vi "SUB_StimGenerator.vi"(0 "SampleNumIn":dbl, 1 "DataFromFile":T2(array[cluster]), 5 "PosInStimTable":i32, 6 "RelativeAmps":bool, 7 "StimType":string, 9 "StimTable":dbl[][](array[numeric]), 11 "UnitFactor":dbl, 12 "SampleRate":dbl, 14 "CommandDivider":dbl) -> (2 "unscaled wave":waveform(dbl), 3 "wave":waveform(dbl), 4 "Array":dbl[](array[numeric]), 10 "Holding":dbl, 13 "UnscaledArray":dbl[](array[numeric]), 15 "SampleNumOut":dbl)   [LabVIEW 2015]
uses:
  <vilib>/Analysis/1siggen.llb/Ramp Pattern by Samples.vi
  <vilib>/Analysis/NI_AALBase.lvlib
panel:
  out "SelCounter":i32
  in  "Cluster":T1={"Pattern"=0, "Mode"=0, "FrameN"=0, "SampleNum"=0, "Flags"=0, "SampleRate"=0.0, "Comment"="", "TimeStr"="", "Data"=[], "StimTable"=[], "NumInFile"=0, "PosInFile"=0, "TimeStamp"=timestamp(0 s since 1904-01-01), "RelAmp"=TRUE}
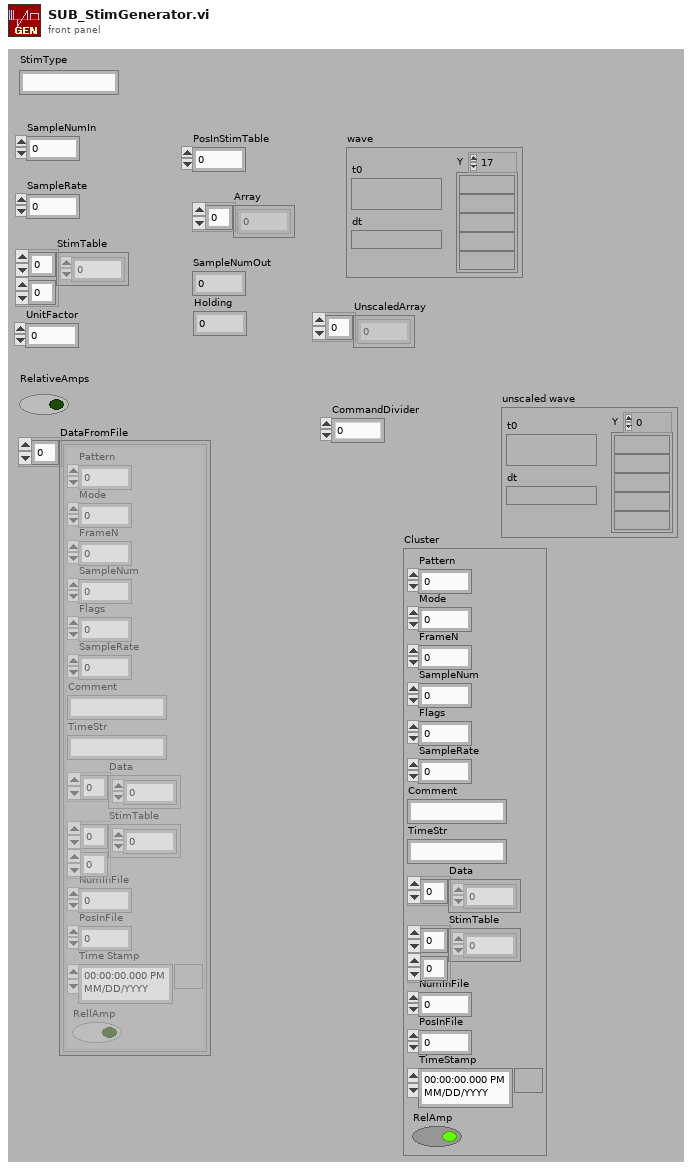
[diagram p1: front panel]
types:
  T1 = cluster{"Pattern":u8, "Mode":u8, "FrameN":u32, "SampleNum":u32, "Flags":u8, "SampleRate":dbl, "Comment":string, "TimeStr":string, "Data":dbl[], "StimTable":dbl[][], "NumInFile":i32, "PosInFile":i32, "TimeStamp":timestamp, "RelAmp":bool}
  T2 = cluster{"Pattern":u8, "Mode":u8, "FrameN":u32, "SampleNum":u32, "Flags":u8, "SampleRate":dbl, "Comment":string, "TimeStr":string, "Data":dbl[], "StimTable":dbl[][], "NumInFile":i32, "PosInFile":i32, "Time Stamp":timestamp, "RellAmp":bool}[]
  T3 = cluster{"Pattern":u8, "Mode":u8, "FrameN":u32, "SampleNum":u32, "Flags":u8, "SampleRate":dbl, "Comment":string, "TimeStr":string, "Data":dbl[], "StimTable":dbl[][], "NumInFile":i32, "PosInFile":i32, "Time Stamp":timestamp, "RellAmp":bool}
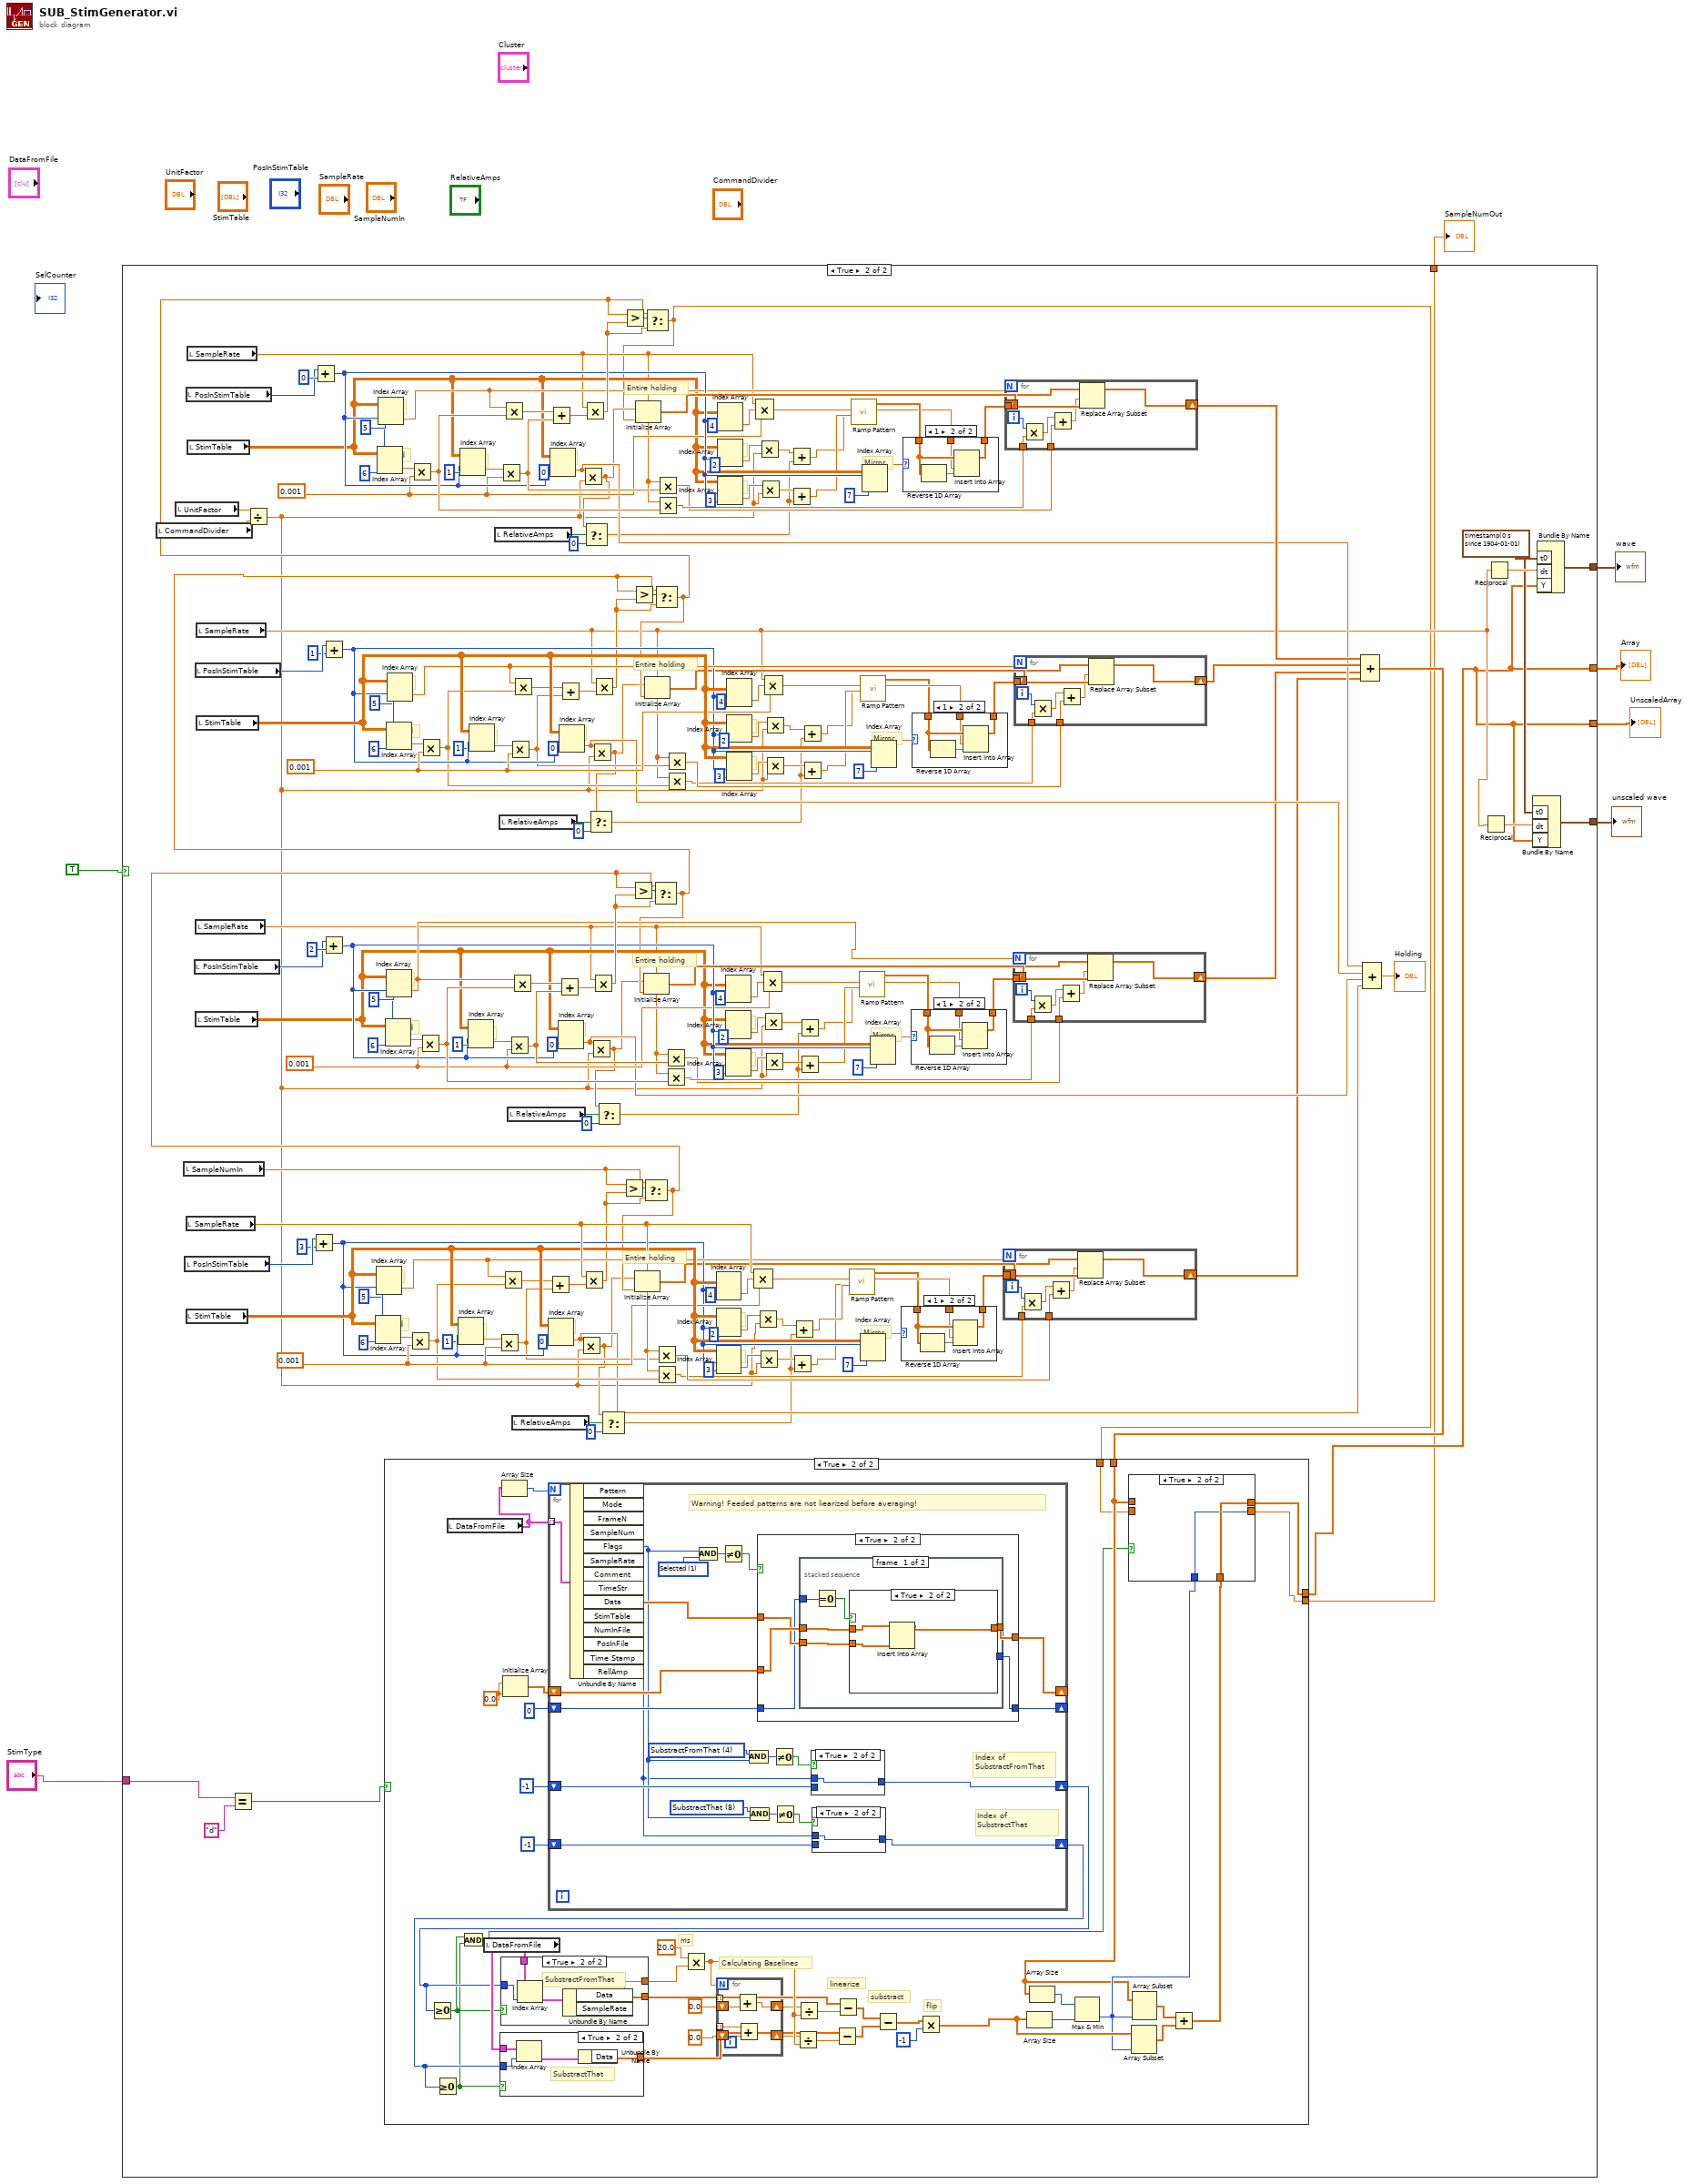
[diagram p0: block diagram]
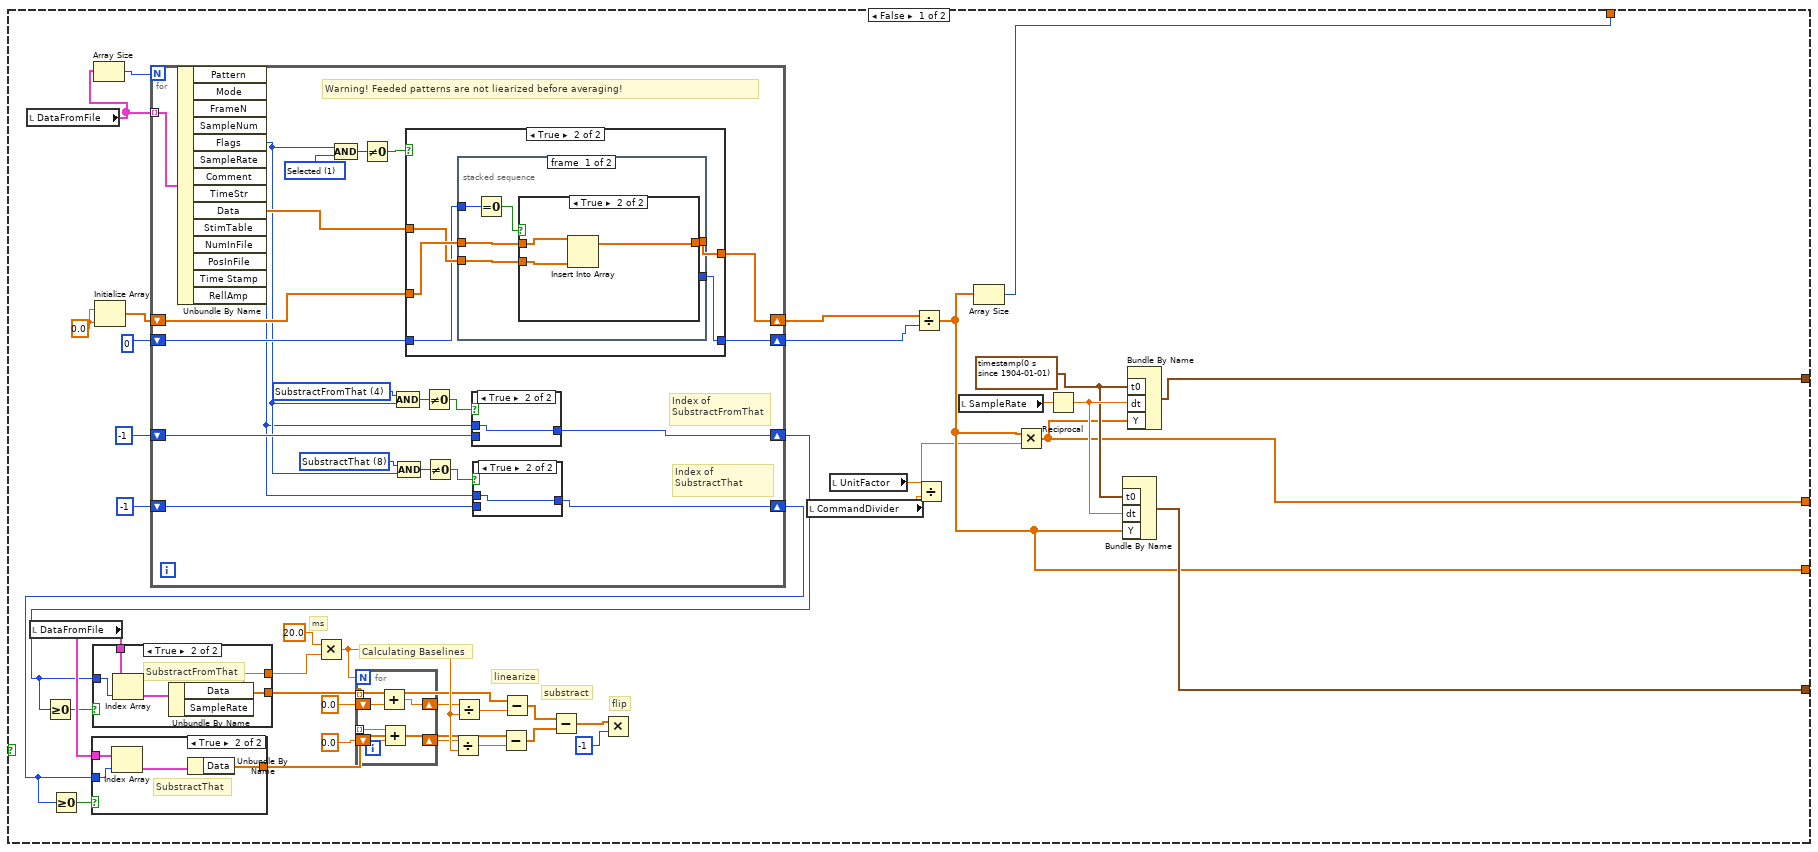
[diagram p2: hidden frame]
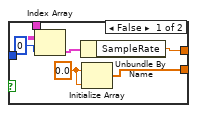
[diagram p3: hidden frame]
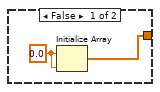
[diagram p4: hidden frame]
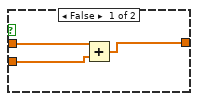
[diagram p8: hidden frame]
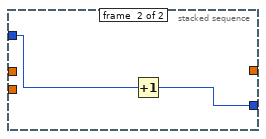
[diagram p9: hidden frame]
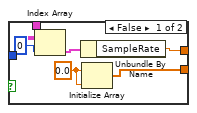
[diagram p12: hidden frame]
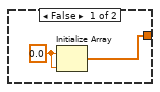
[diagram p13: hidden frame]
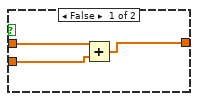
[diagram p17: hidden frame]
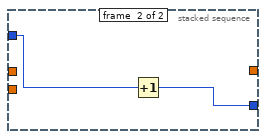
[diagram p18: hidden frame]
diagram:
  n1 = case shown="True" TRUE {
    tunnel: [w35 w119] -> w7
    tunnel: [w40 w130] -> w6
    tunnel: [w44 w129] -> w5
    tunnel: [w34 w121] -> w4
    tunnel: [w39 w121] -> w3
    tunnel: "StimType" -> [_ w116]
    frame False {
      w41 = timestamp(0 s since 1904-01-01)
      w47 = 0.0
      # "flip"
      # "substract"
      # "linearize"
      # "ms"
      # "Calculating Baselines"
      n2 = local read "DataFromFile"() -> (w37:T2)
      n3 = local read "DataFromFile"() -> (w28:T2)
      n4 = Array Size(array=w37) -> (size(s)=w38:i32)
      n5 = Initialize Array(w47, w47) -> (w46:dbl[])
      n6 = for {
        N: w38 -> [_]
        tunnel: w37 -> [w91] mode=indexing
        shift-right: [w85] -> w45
        shift-left: w46 -> [w87]
        shift-right: [w83] -> w36
        shift-left: 0 -> [w84]
        shift-right: [w79] -> w11
        shift-left: -1 -> [w78]
        shift-right: [w71] -> w9
        shift-left: -1 -> [w72]
        w76 = u16 8 items=["Selected"=1, "Deleted"=2, "SubstractFromThat"=4, "SubstractThat"=8] ("DataFrameFlags")
        w81 = u16 4 items=["Selected"=1, "Deleted"=2, "SubstractFromThat"=4, "SubstractThat"=8] ("DataFrameFlags")
        w90 = u16 1 items=["Selected"=1, "Deleted"=2, "Reserved1"=4, "Reserved2"=8] ("DataFrameFlags")
        # "Index of SubstractThat"
        # "Index of SubstractFromThat"
        # "Warning! Feeded patterns are not liearized before averaging!"
        n7 = Unbundle By Name(w91) -> ("Flags"=w74:u8, "Data"=w86:dbl[], "NumInFile"=w73:i32)  [unwired: 11 out]
        n8 = Compound Arithmetic op=AND(w74, w90) -> (w89:u16)
        n9 = Not Equal To 0?(x=w89) -> (x != 0?=w88:bool)
        n10 = Compound Arithmetic op=AND(w81, w74) -> (w82:u16)
        n11 = Compound Arithmetic op=AND(w76, w74) -> (w75:u16)
        n12 = case shown="True" w88 {
          tunnel: w87 -> [w97 w102]
          tunnel: [w97 w100] -> w85
          tunnel: w86 -> [_ w101]
          tunnel: w84 -> [w96 w99]
          tunnel: [w96 w98] -> w83
          frame False {
          }
          frame True {
            n13 = stacked-sequence {
              tunnel: w102 -> [w107 _]
              tunnel: w101 -> [w106 _]
              tunnel: [w105 _] -> w100
              tunnel: w99 -> [w103 w115]
              tunnel: [_ w114] -> w98
              frame #0 {
                n14 = Equal To 0?(x=w103) -> (x = 0?=w104:bool)
                n15 = case shown="True" w104 {
                  tunnel: w107 -> [w109 w112]
                  tunnel: w106 -> [w110 w111]
                  tunnel: [w108 w113] -> w105
                  frame False {
                    n16 = Add(x=w109, y=w110) -> (x+y=w108:dbl[])
                  }
                  frame True {
                    n17 = Insert Into Array(array=w112, new element=w111) -> (w113:dbl[])  [unwired: 1 in]
                  }
                }
              }
              frame #1 {
                n18 = Increment(x=w115) -> (x+1=w114:i32)
              }
            }
          }
        }
        n19 = Not Equal To 0?(x=w82) -> (x != 0?=w80:bool)
        n20 = Not Equal To 0?(x=w75) -> (x != 0?=w77:bool)
        n21 = case shown="True" w80 {
          tunnel: w73 -> [_ w95]
          tunnel: [w94 w95] -> w79
          tunnel: w78 -> [w94 _]
          frame False {
          }
          frame True {
          }
        }
        n22 = case shown="True" w77 {
          tunnel: w73 -> [_ w93]
          tunnel: [w92 w93] -> w71
          tunnel: w72 -> [w92 _]
          frame False {
          }
          frame True {
          }
        }
      }
      n23 = Greater Or Equal To 0?(x=w11) -> (x >= 0?=w12:bool)
      n24 = Greater Or Equal To 0?(x=w9) -> (x >= 0?=w10:bool)
      n25 = case shown="True" w10 {
        tunnel: w28 -> [_ w64]
        tunnel: w9 -> [_ w63]
        tunnel: [w59 w61] -> w17
        frame False {
          w60 = 0.0
          n26 = Initialize Array(w60, w60) -> (w59:dbl[])
        }
        frame True {
          # "SubstractThat"
          n27 = Index Array(array=w64, index=w63) -> (element=w62:T3)
          n28 = Unbundle By Name(w62) -> ("Data"=w61:dbl[])
        }
      }
      n29 = case shown="True" w12 {
        tunnel: w11 -> [_ w58]
        tunnel: w28 -> [w52 w57]
        tunnel: [w50 w55] -> w26
        tunnel: [w49 w54] -> w19
        frame False {
          w48 = 0.0
          n30 = Index Array(array=w52, index=0) -> (element=w53:T3)
          n31 = Unbundle By Name(w53) -> ("SampleRate"=w50:dbl)
          n32 = Initialize Array(w48, w48) -> (w49:dbl[])
        }
        frame True {
          # "SubstractFromThat"
          n33 = Index Array(array=w57, index=w58) -> (element=w56:T3)
          n34 = Unbundle By Name(w56) -> ("Data"=w54:dbl[], "SampleRate"=w55:dbl)
        }
      }
      n35 = Multiply(x=20.0, y=w26) -> (x*y=w23:dbl)
      n36 = for {
        N: w23 -> [_]
        tunnel: w19 -> [w69] mode=indexing
        tunnel: w17 -> [w66] mode=indexing
        shift-right: [w68] -> w22
        shift-left: 0.0 -> [w70]
        shift-right: [w65] -> w21
        shift-left: 0.0 -> [w67]
        n37 = Add(x=w69, y=w70) -> (x+y=w68:dbl)
        n38 = Add(x=w66, y=w67) -> (x+y=w65:dbl)
      }
      n39 = Divide(x=w21, y=w23) -> (x/y=w18:dbl)
      n40 = Divide(x=w22, y=w23) -> (x/y=w20:dbl)
      n41 = Subtract(x=w17, y=w18) -> (x-y=w15:dbl[])
      n42 = Subtract(x=w19, y=w20) -> (x-y=w16:dbl[])
      n43 = Subtract(x=w16, y=w15) -> (x-y=w14:dbl[])
      n44 = Multiply(x=w14, y=-1) -> ()  [unwired: 1 out]
      n45 = local read "CommandDivider"() -> (w33:dbl)
      n46 = local read "UnitFactor"() -> (w32:dbl)
      n47 = Divide(x=w45, y=w36) -> (x/y=w34:dbl[])
      n48 = Divide(x=w32, y=w33) -> (x/y=w31:dbl)
      n49 = local read "SampleRate"() -> (w43:dbl)
      n50 = Array Size(array=w34) -> (size(s)=w35:i32)
      n51 = Multiply(x=w34, y=w31) -> (x*y=w39:dbl[])
      n52 = Reciprocal(x=w43) -> (1/x=w42:dbl)
      n53 = Bundle By Name("t0"=w41, "dt"=w42, "Y"=w34) -> (w44:waveform(dbl))  [unwired: 1 out]
      n54 = Bundle By Name("t0"=w41, "dt"=w42, "Y"=w39) -> (w40:waveform(dbl))  [unwired: 1 out]
    }
    frame True {
      w126 = timestamp(0 s since 1904-01-01)
      w194 = 0.001
      w209 = 0.001
      w270 = 0.001
      w280 = 0.001
      # "Mirror"
      # "Amp2"
      # "Amp1"
      # "Dur"
      # "Hold"
      # "Delay"
      # "Entire holding"
      # "Period"
      # "Num"
      # "Mirror"
      # "Amp2"
      # "Amp1"
      # "Dur"
      # "Hold"
      # "Delay"
      # "Entire holding"
      # "Period"
      # "Num"
      # "Mirror"
      # "Amp2"
      # "Amp1"
      # "Dur"
      # "Hold"
      # "Delay"
      # "Entire holding"
      # "Period"
      # "Num"
      # "Mirror"
      # "Amp2"
      # "Amp1"
      # "Dur"
      # "Hold"
      # "Delay"
      # "Entire holding"
      # "Period"
      # "Num"
      n55 = local read "CommandDivider"() -> (w125:dbl)
      n56 = local read "UnitFactor"() -> (w124:dbl)
      n57 = local read "SampleNumIn"() -> (w200:dbl)
      n58 = local read "PosInStimTable"() -> (w198:i32)
      n59 = local read "PosInStimTable"() -> (w276:i32)
      n60 = local read "SampleRate"() -> (w199:dbl)
      n61 = local read "StimTable"() -> (w197:dbl[][])
      n62 = local read "SampleRate"() -> (w275:dbl)
      n63 = local read "StimTable"() -> (w277:dbl[][])
      n64 = local read "PosInStimTable"() -> (w205:i32)
      n65 = local read "PosInStimTable"() -> (w274:i32)
      n66 = local read "SampleRate"() -> (w204:dbl)
      n67 = local read "StimTable"() -> (w206:dbl[][])
      n68 = local read "SampleRate"() -> (w127:dbl)
      n69 = local read "StimTable"() -> (w273:dbl[][])
      n70 = Equal?(x=w116, y="d") -> (x = y?=w117:bool)
      n71 = Divide(x=w124, y=w125) -> (x/y=w123:dbl)
      n72 = Add(x=w198, y=3) -> (x+y=w192:i32)
      n73 = Add(x=w276, y=0) -> (x+y=w282:i32)
      n74 = Add(x=w205, y=2) -> (x+y=w211:i32)
      n75 = Add(x=w274, y=1) -> (x+y=w268:i32)
      n76 = Index Array(array=w197, index (row)=w192, index (col)=6) -> (element=w188:dbl)
      n77 = Index Array(array=w197, index (row)=w192, index (col)=5) -> (element=w193:dbl)
      n78 = Index Array(array=w277, index (row)=w282, index (col)=6) -> (element=w286:dbl)
      n79 = Index Array(array=w277, index (row)=w282, index (col)=5) -> (element=w281:dbl)
      n80 = Index Array(array=w206, index (row)=w211, index (col)=6) -> (element=w215:dbl)
      n81 = Index Array(array=w273, index (row)=w268, index (col)=6) -> (element=w264:dbl)
      n82 = Index Array(array=w206, index (row)=w211, index (col)=5) -> (element=w210:dbl)
      n83 = Index Array(array=w273, index (row)=w268, index (col)=5) -> (element=w269:dbl)
      n84 = Multiply(x=w188, y=w194) -> (x*y=w189:dbl)
      n85 = Multiply(x=w286, y=w280) -> (x*y=w285:dbl)
      n86 = Multiply(x=w215, y=w209) -> (x*y=w214:dbl)
      n87 = Multiply(x=w264, y=w270) -> (x*y=w265:dbl)
      n88 = Index Array(array=w197, index (row)=w192, index (col)=1) -> (element=w191:dbl)
      n89 = Index Array(array=w277, index (row)=w282, index (col)=1) -> (element=w283:dbl)
      n90 = Index Array(array=w206, index (row)=w211, index (col)=1) -> (element=w212:dbl)
      n91 = Index Array(array=w273, index (row)=w268, index (col)=1) -> (element=w267:dbl)
      n92 = local read "RelativeAmps"() -> (w163:bool)
      n93 = Multiply(x=w191, y=w194) -> (x*y=w190:dbl)
      n94 = Multiply(x=w283, y=w280) -> (x*y=w284:dbl)
      n95 = local read "RelativeAmps"() -> (w154:bool)
      n96 = Multiply(x=w193, y=w189) -> (x*y=w178:dbl)
      n97 = Multiply(x=w281, y=w285) -> (x*y=w296:dbl)
      n98 = Multiply(x=w212, y=w209) -> (x*y=w213:dbl)
      n99 = Multiply(x=w267, y=w270) -> (x*y=w266:dbl)
      n100 = local read "RelativeAmps"() -> (w147:bool)
      n101 = Multiply(x=w210, y=w214) -> (x*y=w225:dbl)
      n102 = Multiply(x=w269, y=w265) -> (x*y=w254:dbl)
      n103 = local read "RelativeAmps"() -> (w138:bool)
      n104 = Add(x=w178, y=w190) -> (x+y=w177:dbl)
      n105 = Index Array(array=w197, index (row)=w192, index (col)=0) -> (element=w164:dbl)
      n106 = Add(x=w296, y=w284) -> (x+y=w297:dbl)
      n107 = Index Array(array=w277, index (row)=w282, index (col)=0) -> (element=w239:dbl)
      n108 = Add(x=w225, y=w213) -> (x+y=w226:dbl)
      n109 = Add(x=w254, y=w266) -> (x+y=w253:dbl)
      n110 = Index Array(array=w206, index (row)=w211, index (col)=0) -> (element=w201:dbl)
      n111 = Index Array(array=w273, index (row)=w268, index (col)=0) -> (element=w238:dbl)
      n112 = Multiply(x=w164, y=w123) -> (x*y=w137:dbl)
      n113 = Multiply(x=w239, y=w123) -> (x*y=w161:dbl)
      n114 = Multiply(x=w199, y=w177) -> (x*y=w168:dbl)
      n115 = Multiply(x=w275, y=w297) -> (x*y=w306:dbl)
      n116 = Select(t=w161, s=w163, f=0) -> (s? t:f=w156:dbl)
      n117 = Multiply(x=w201, y=w123) -> (x*y=w145:dbl)
      n118 = Multiply(x=w238, y=w123) -> (x*y=w153:dbl)
      n119 = Select(t=w153, s=w154, f=0) -> (s? t:f=w148:dbl)
      n120 = Multiply(x=w204, y=w226) -> (x*y=w235:dbl)
      n121 = Multiply(x=w127, y=w253) -> (x*y=w244:dbl)
      n122 = Select(t=w145, s=w147, f=0) -> (s? t:f=w140:dbl)
      n123 = Select(t=w137, s=w138, f=0) -> (s? t:f=w132:dbl)
      n124 = Greater?(x=w200, y=w168) -> (0:w167:bool)
      n125 = Select(t=w200, s=w167, f=w168) -> (s? t:f=w166:dbl)
      n126 = Greater?(x=w166, y=w235) -> (0:w236:bool)
      n127 = Initialize Array(w137, w166) -> (w175:dbl[])
      n128 = Select(t=w166, s=w236, f=w235) -> (s? t:f=w203:dbl)
      n129 = Greater?(x=w203, y=w244) -> (0:w243:bool)
      n130 = Initialize Array(w145, w203) -> (w228:dbl[])
      n131 = Select(t=w203, s=w243, f=w244) -> (s? t:f=w240:dbl)
      n132 = Greater?(x=w240, y=w306) -> (0:w307:bool)
      n133 = Select(t=w240, s=w307, f=w306) -> (s? t:f=w120:dbl)
      n134 = Initialize Array(w161, w120) -> (w299:dbl[])
      n135 = Initialize Array(w153, w240) -> (w251:dbl[])
      n136 = Multiply(x=w199, y=w190) -> (x*y=w170:dbl)
      n137 = Multiply(x=w199, y=w189) -> (x*y=w169:dbl)
      n138 = Multiply(x=w275, y=w284) -> (x*y=w304:dbl)
      n139 = Multiply(x=w275, y=w285) -> (x*y=w305:dbl)
      n140 = Multiply(x=w204, y=w213) -> (x*y=w233:dbl)
      n141 = Multiply(x=w204, y=w214) -> (x*y=w234:dbl)
      n142 = Multiply(x=w127, y=w266) -> (x*y=w246:dbl)
      n143 = Multiply(x=w127, y=w265) -> (x*y=w245:dbl)
      n144 = Index Array(array=w197, index (row)=w192, index (col)=4) -> (element=w172:dbl)
      n145 = Index Array(array=w197, index (row)=w192, index (col)=2) -> (element=w196:dbl)
      n146 = Index Array(array=w197, index (row)=w192, index (col)=3) -> (element=w195:dbl)
      n147 = Index Array(array=w277, index (row)=w282, index (col)=4) -> (element=w302:dbl)
      n148 = Index Array(array=w277, index (row)=w282, index (col)=2) -> (element=w278:dbl)
      n149 = Index Array(array=w277, index (row)=w282, index (col)=3) -> (element=w279:dbl)
      n150 = Index Array(array=w206, index (row)=w211, index (col)=4) -> (element=w231:dbl)
      n151 = Index Array(array=w206, index (row)=w211, index (col)=2) -> (element=w207:dbl)
      n152 = Index Array(array=w206, index (row)=w211, index (col)=3) -> (element=w208:dbl)
      n153 = Index Array(array=w273, index (row)=w268, index (col)=4) -> (element=w248:dbl)
      n154 = Index Array(array=w273, index (row)=w268, index (col)=2) -> (element=w272:dbl)
      n155 = Index Array(array=w273, index (row)=w268, index (col)=3) -> (element=w271:dbl)
      n156 = Compound Arithmetic op=MULTIPLY(w199, w172, w194) -> (w183:dbl)
      n157 = Compound Arithmetic op=MULTIPLY(w275, w302, w280) -> (w291:dbl)
      n158 = Multiply(x=w196, y=w123) -> (x*y=w135:dbl)
      n159 = Multiply(x=w195, y=w123) -> (x*y=w133:dbl)
      n160 = Multiply(x=w278, y=w123) -> (x*y=w157:dbl)
      n161 = Multiply(x=w279, y=w123) -> (x*y=w159:dbl)
      n162 = Multiply(x=w207, y=w123) -> (x*y=w142:dbl)
      n163 = Multiply(x=w208, y=w123) -> (x*y=w141:dbl)
      n164 = Multiply(x=w272, y=w123) -> (x*y=w149:dbl)
      n165 = Multiply(x=w271, y=w123) -> (x*y=w151:dbl)
      n166 = Compound Arithmetic op=MULTIPLY(w204, w231, w209) -> (w220:dbl)
      n167 = Compound Arithmetic op=MULTIPLY(w127, w248, w270) -> (w259:dbl)
      n168 = Add(x=w157, y=w156) -> (x+y=w158:dbl)
      n169 = Add(x=w159, y=w156) -> (x+y=w160:dbl)
      n170 = Add(x=w133, y=w132) -> (x+y=w134:dbl)
      n171 = Add(x=w135, y=w132) -> (x+y=w136:dbl)
      n172 = Add(x=w142, y=w140) -> (x+y=w143:dbl)
      n173 = Add(x=w141, y=w140) -> (x+y=w144:dbl)
      n174 = Add(x=w149, y=w148) -> (x+y=w150:dbl)
      n175 = Add(x=w151, y=w148) -> (x+y=w152:dbl)
      n176 = call-poly <vilib>:"Ramp Pattern.vi"("start"=w136, "end"=w134, "samples"=w183) -> ("Ramp Pattern"=w182:dbl[])  [unwired: 7 in, 1 out]
      n177 = call-poly <vilib>:"Ramp Pattern.vi"("start"=w158, "end"=w160, "samples"=w291) -> ("Ramp Pattern"=w292:dbl[])  [unwired: 7 in, 1 out]
      n178 = call-poly <vilib>:"Ramp Pattern.vi"("start"=w143, "end"=w144, "samples"=w220) -> ("Ramp Pattern"=w221:dbl[])  [unwired: 7 in, 1 out]
      n179 = call-poly <vilib>:"Ramp Pattern.vi"("start"=w150, "end"=w152, "samples"=w259) -> ("Ramp Pattern"=w258:dbl[])  [unwired: 7 in, 1 out]
      n180 = Index Array(array=w197, index (row)=w192, index (col)=7) -> (element=w187:dbl)
      n181 = Index Array(array=w277, index (row)=w282, index (col)=7) -> (element=w287:dbl)
      n182 = Index Array(array=w206, index (row)=w211, index (col)=7) -> (element=w216:dbl)
      n183 = Index Array(array=w273, index (row)=w268, index (col)=7) -> (element=w263:dbl)
      n184 = case shown="1" w187 {
        tunnel: w182 -> [w421 w425]
        tunnel: w183 -> [_ w423]
        tunnel: [w421 w422] -> w184
        frame 0, Default {
        }
        frame 1 {
          n185 = Reverse 1D Array(array=w425) -> (reversed array=w424:dbl[])
          n186 = Insert Into Array(array=w425, index=w423, new element=w424) -> (w422:dbl[])
        }
      }
      n187 = case shown="1" w287 {
        tunnel: w292 -> [w460 w464]
        tunnel: w291 -> [_ w462]
        tunnel: [w460 w461] -> w290
        frame 0, Default {
        }
        frame 1 {
          n188 = Reverse 1D Array(array=w464) -> (reversed array=w463:dbl[])
          n189 = Insert Into Array(array=w464, index=w462, new element=w463) -> (w461:dbl[])
        }
      }
      n190 = case shown="1" w216 {
        tunnel: w221 -> [w434 w438]
        tunnel: w220 -> [_ w436]
        tunnel: [w434 w435] -> w219
        frame 0, Default {
        }
        frame 1 {
          n191 = Reverse 1D Array(array=w438) -> (reversed array=w437:dbl[])
          n192 = Insert Into Array(array=w438, index=w436, new element=w437) -> (w435:dbl[])
        }
      }
      n193 = case shown="1" w263 {
        tunnel: w258 -> [w447 w451]
        tunnel: w259 -> [_ w449]
        tunnel: [w447 w448] -> w260
        frame 0, Default {
        }
        frame 1 {
          n194 = Reverse 1D Array(array=w451) -> (reversed array=w450:dbl[])
          n195 = Insert Into Array(array=w451, index=w449, new element=w450) -> (w448:dbl[])
        }
      }
      n196 = for {
        N: w193 -> [_]
        shift-right: [w426] -> w165
        shift-left: w175 -> [w433]
        tunnel: w184 -> [w432]
        tunnel: w170 -> [w429]
        tunnel: w169 -> [w428]
        i -> [w427]
        n197 = Multiply(x=w427, y=w428) -> (x*y=w430:dbl)
        n198 = Add(x=w430, y=w429) -> (x+y=w431:dbl)
        n199 = Replace Array Subset(array=w433, new element=w432, index=w431) -> (w426:dbl[])
      }
      n200 = for {
        N: w281 -> [_]
        shift-right: [w465] -> w242
        shift-left: w299 -> [w472]
        tunnel: w290 -> [w471]
        tunnel: w304 -> [w468]
        tunnel: w305 -> [w467]
        i -> [w466]
        n201 = Multiply(x=w466, y=w467) -> (x*y=w469:dbl)
        n202 = Add(x=w469, y=w468) -> (x+y=w470:dbl)
        n203 = Replace Array Subset(array=w472, new element=w471, index=w470) -> (w465:dbl[])
      }
      n204 = for {
        N: w210 -> [_]
        shift-right: [w439] -> w202
        shift-left: w228 -> [w446]
        tunnel: w219 -> [w445]
        tunnel: w233 -> [w442]
        tunnel: w234 -> [w441]
        i -> [w440]
        n205 = Multiply(x=w440, y=w441) -> (x*y=w443:dbl)
        n206 = Add(x=w443, y=w442) -> (x+y=w444:dbl)
        n207 = Replace Array Subset(array=w446, new element=w445, index=w444) -> (w439:dbl[])
      }
      n208 = for {
        N: w269 -> [_]
        shift-right: [w452] -> w241
        shift-left: w251 -> [w459]
        tunnel: w260 -> [w458]
        tunnel: w246 -> [w455]
        tunnel: w245 -> [w454]
        i -> [w453]
        n209 = Multiply(x=w453, y=w454) -> (x*y=w456:dbl)
        n210 = Add(x=w456, y=w455) -> (x+y=w457:dbl)
        n211 = Replace Array Subset(array=w459, new element=w458, index=w457) -> (w452:dbl[])
      }
      n212 = Compound Arithmetic op=ADD(w242, w241, w202, w165) -> (w122:dbl[])
      n213 = case shown="True" w117 {
        tunnel: w122 -> [w309 w314]
        tunnel: [w309 w318] -> w121
        tunnel: w120 -> [w308 w313]
        tunnel: [w308 w317] -> w119
        frame False {
        }
        frame True {
          w348 = 0.0
          # "flip"
          # "substract"
          # "linearize"
          # "ms"
          # "Calculating Baselines"
          n214 = local read "DataFromFile"() -> (w345:T2)
          n215 = local read "DataFromFile"() -> (w342:T2)
          n216 = Array Size(array=w345) -> (size(s)=w346:i32)
          n217 = Initialize Array(w348, w348) -> (w347:dbl[])
          n218 = for {
            N: w346 -> [_]
            tunnel: w345 -> [w396] mode=indexing
            shift-right: [w390] -> _
            shift-left: w347 -> [w392]
            shift-right: [w388] -> _
            shift-left: 0 -> [w389]
            shift-right: [w384] -> w326
            shift-left: -1 -> [w383]
            shift-right: [w376] -> w325
            shift-left: -1 -> [w377]
            w381 = u16 8 items=["Selected"=1, "Deleted"=2, "SubstractFromThat"=4, "SubstractThat"=8] ("DataFrameFlags")
            w386 = u16 4 items=["Selected"=1, "Deleted"=2, "SubstractFromThat"=4, "SubstractThat"=8] ("DataFrameFlags")
            w395 = u16 1 items=["Selected"=1, "Deleted"=2, "Reserved1"=4, "Reserved2"=8] ("DataFrameFlags")
            # "Index of SubstractThat"
            # "Index of SubstractFromThat"
            # "Warning! Feeded patterns are not liearized before averaging!"
            n219 = Unbundle By Name(w396) -> ("Flags"=w379:u8, "Data"=w391:dbl[], "NumInFile"=w378:i32)  [unwired: 11 out]
            n220 = Compound Arithmetic op=AND(w379, w395) -> (w394:u16)
            n221 = Not Equal To 0?(x=w394) -> (x != 0?=w393:bool)
            n222 = Compound Arithmetic op=AND(w386, w379) -> (w387:u16)
            n223 = Compound Arithmetic op=AND(w381, w379) -> (w380:u16)
            n224 = case shown="True" w393 {
              tunnel: w392 -> [w402 w407]
              tunnel: [w402 w405] -> w390
              tunnel: w391 -> [_ w406]
              tunnel: w389 -> [w401 w404]
              tunnel: [w401 w403] -> w388
              frame False {
              }
              frame True {
                n225 = stacked-sequence {
                  tunnel: w407 -> [w412 _]
                  tunnel: w406 -> [w411 _]
                  tunnel: [w410 _] -> w405
                  tunnel: w404 -> [w408 w420]
                  tunnel: [_ w419] -> w403
                  frame #0 {
                    n226 = Equal To 0?(x=w408) -> (x = 0?=w409:bool)
                    n227 = case shown="True" w409 {
                      tunnel: w412 -> [w414 w417]
                      tunnel: w411 -> [w415 w416]
                      tunnel: [w413 w418] -> w410
                      frame False {
                        n228 = Add(x=w414, y=w415) -> (x+y=w413:dbl[])
                      }
                      frame True {
                        n229 = Insert Into Array(array=w417, new element=w416) -> (w418:dbl[])  [unwired: 1 in]
                      }
                    }
                  }
                  frame #1 {
                    n230 = Increment(x=w420) -> (x+1=w419:i32)
                  }
                }
              }
            }
            n231 = Not Equal To 0?(x=w387) -> (x != 0?=w385:bool)
            n232 = Not Equal To 0?(x=w380) -> (x != 0?=w382:bool)
            n233 = case shown="True" w385 {
              tunnel: w378 -> [_ w400]
              tunnel: [w399 w400] -> w384
              tunnel: w383 -> [w399 _]
              frame False {
              }
              frame True {
              }
            }
            n234 = case shown="True" w382 {
              tunnel: w378 -> [_ w398]
              tunnel: [w397 w398] -> w376
              tunnel: w377 -> [w397 _]
              frame False {
              }
              frame True {
              }
            }
          }
          n235 = Greater Or Equal To 0?(x=w326) -> (x >= 0?=w312:bool)
          n236 = Greater Or Equal To 0?(x=w325) -> (x >= 0?=w311:bool)
          n237 = And(x=w312, y=w311) -> (x .and. y?=w310:bool)
          n238 = case shown="True" w311 {
            tunnel: w342 -> [_ w369]
            tunnel: w325 -> [_ w368]
            tunnel: [w364 w366] -> w331
            frame False {
              w365 = 0.0
              n239 = Initialize Array(w365, w365) -> (w364:dbl[])
            }
            frame True {
              # "SubstractThat"
              n240 = Index Array(array=w369, index=w368) -> (element=w367:T3)
              n241 = Unbundle By Name(w367) -> ("Data"=w366:dbl[])
            }
          }
          n242 = case shown="True" w312 {
            tunnel: w326 -> [_ w363]
            tunnel: w342 -> [w357 w362]
            tunnel: [w355 w360] -> w340
            tunnel: [w354 w359] -> w333
            frame False {
              w353 = 0.0
              n243 = Index Array(array=w357, index=0) -> (element=w358:T3)
              n244 = Unbundle By Name(w358) -> ("SampleRate"=w355:dbl)
              n245 = Initialize Array(w353, w353) -> (w354:dbl[])
            }
            frame True {
              # "SubstractFromThat"
              n246 = Index Array(array=w362, index=w363) -> (element=w361:T3)
              n247 = Unbundle By Name(w361) -> ("Data"=w359:dbl[], "SampleRate"=w360:dbl)
            }
          }
          n248 = Multiply(x=20.0, y=w340) -> (x*y=w337:dbl)
          n249 = for {
            N: w337 -> [_]
            tunnel: w333 -> [w374] mode=indexing
            tunnel: w331 -> [w371] mode=indexing
            shift-right: [w373] -> w336
            shift-left: 0.0 -> [w375]
            shift-right: [w370] -> w335
            shift-left: 0.0 -> [w372]
            n250 = Add(x=w374, y=w375) -> (x+y=w373:dbl)
            n251 = Add(x=w371, y=w372) -> (x+y=w370:dbl)
          }
          n252 = Divide(x=w335, y=w337) -> (x/y=w332:dbl)
          n253 = Divide(x=w336, y=w337) -> (x/y=w334:dbl)
          n254 = Subtract(x=w331, y=w332) -> (x-y=w329:dbl[])
          n255 = Subtract(x=w333, y=w334) -> (x-y=w330:dbl[])
          n256 = Subtract(x=w330, y=w329) -> (x-y=w328:dbl[])
          n257 = Multiply(x=w328, y=-1) -> (x*y=w321:dbl[])
          n258 = Array Size(array=w321) -> (size(s)=w323:i32)
          n259 = Array Size(array=w314) -> (size(s)=w322:i32)
          n260 = Max & Min(x=w322, y=w323) -> (min(x,y)=w315:i32)  [unwired: 1 out]
          n261 = Array Subset(array=w321, length=w315) -> (w320:dbl[])  [unwired: 1 in]
          n262 = Array Subset(array=w314, length=w315) -> (w319:dbl[])  [unwired: 1 in]
          n263 = Add(x=w319, y=w320) -> (x+y=w316:dbl[])
          n264 = case shown="True" w310 {
            tunnel: [w350 w352] -> w318
            tunnel: [w349 w351] -> w317
            tunnel: w316 -> [_ w352]
            tunnel: w315 -> [_ w351]
            tunnel: w314 -> [w350 _]
            tunnel: w313 -> [w349 _]
            frame False {
            }
            frame True {
            }
          }
        }
      }
      n265 = Compound Arithmetic op=ADD(w239, w238, w201, w164) -> (→"Holding":dbl)
      n266 = Reciprocal(x=w127) -> (1/x=w128:dbl)
      n267 = Reciprocal(x=w127) -> (1/x=w131:dbl)
      n268 = Bundle By Name("t0"=w126, "dt"=w128, "Y"=w121) -> (w129:waveform(dbl))  [unwired: 1 out]
      n269 = Bundle By Name("t0"=w126, "dt"=w131, "Y"=w121) -> (w130:waveform(dbl))  [unwired: 1 out]
    }
  }
  "SampleNumOut" <- w7
  "wave" <- w6
  "unscaled wave" <- w5
  "UnscaledArray" <- w4
  "Array" <- w3
